vi "Quick Usb Write Fpga Data.vi"(8 "error in (no error)":errorcluster, 9 "datalength":u32, 10 "fpgadata":string, 11 "hDevice":u32) -> (0 "error out":errorcluster, 1 "function return":i32, 2 "fpgadata out":string, 3 "hDevice out":u32)   [LabVIEW 2011, in "QuickUSB.lvlib"]
doc: "QUSBLIB QRETURN QuickUsbWriteFpgaData(\n QHANDLE hDevice, \n PQBYTE fpgadata, \n QULONG datalength\n);"
uses:
  QuickUSB.lvlib
  QuickUSB.dll
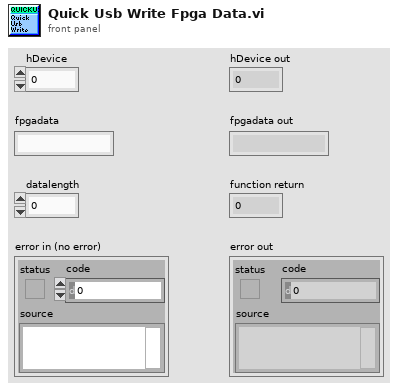
[diagram p1: front panel]
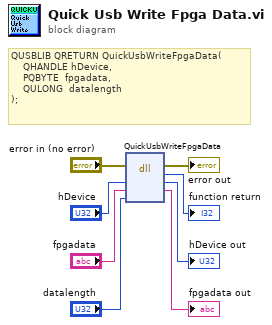
[diagram p0: block diagram]
diagram:
  # "QUSBLIB QRETURN QuickUsbWriteFpgaData(\n    QHANDLE hDevice, \n    PQBYTE  fpgadata, \n    QULONG  datalength\n);"
  n1 = dll-call lib="C:/QuickUSB/QuickUSB.*" fn="QuickUsbWriteFpgaData"(error in="error in (no error)", "hDevice"="hDevice", "fpgadata"="fpgadata", "datalength"="datalength") -> (error out=→"error out":errorcluster, →"function return":i32, "hDevice"=→"hDevice out":u32, "fpgadata"=→"fpgadata out":string)  [unwired: 3 in, 1 out]
